vi "WriteSetting 32bit.vi"(7 "value":u32, 8 "error in (no error)":errorcluster, 10 "FPGA Setting":T1, 11 "FpgaRefBase in":refnum<class "FpgaRefBase.lvclass">) -> (0 "error out":errorcluster, 3 "FpgaRefBase out":refnum<class "FpgaRefBase.lvclass">)   [LabVIEW 2018, in "FpgaRefBase.lvclass"]
uses:
  FpgaRefBase.lvclass
  FPGA/fpga_settings.ctl
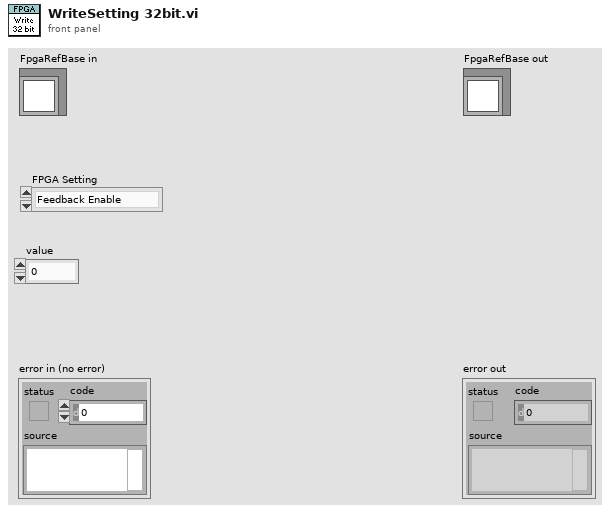
[diagram p1: front panel]
types:
  T1 = typedef "fpga_settings.ctl" = enum16{"Feedback Enable", "New FIR coeffs", "FIR shift", "Enable filter", "Set Downsample", "Downsample", "CIC Gain", "Record length", "Trigger samples", "Quiet time", "a_am", "b_am", "Use fixed delay", "fixed sin_fi", "fixed cos_fi", "Ki*Tau", "Kp", "Kd_Tau", "Fi_start", "Fi_delta", "DC_offs 0", "DC_offs 1", "DC_offs 2", "DC_offs 3", "Ki*Tau am", "Kp am", "Kd_Tau am", "Feedback AM", "Trigger delay", "Feedback delay", "Setpoint enable", "Beam enable", "Samples to acquire", "Cavity Enable", "Cavity C1", "Cavity C2", "Cavity C3", "Cavity C4", "Cavity C5"}
  T2 = typedef "settingsFPGAref.ctl" = refnum<k20>
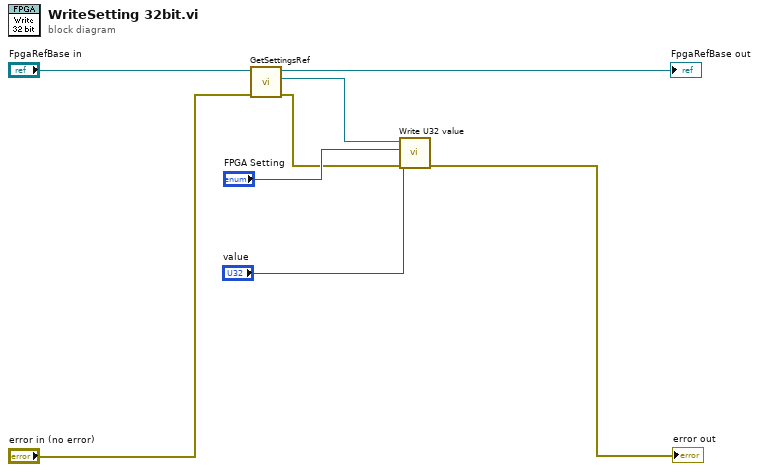
[diagram p0: block diagram]
diagram:
  n1 = call-dynamic "GetSettingsRef.vi"("error in (no error)"="error in (no error)", "FpgaRefBase in"="FpgaRefBase in") -> ("error out"=w1:errorcluster, "Settings FPGA ref"=w4:T2, "FpgaRefBase out"=→"FpgaRefBase out":refnum<class "FpgaRefBase.lvclass">)  [unwired: 7 in]
  n2 = call "Write U32 value.vi"("error in"=w1, "value"="value", "FPGA Setting"="FPGA Setting", "FPGA ref"=w4) -> ("error out"=→"error out":errorcluster)  [unwired: 6 in, 1 out]
